vi "串口助手.vi"() -> ()   [LabVIEW 2012]
uses:
  <vilib>/Instr/_visa.llb/VISA Configure Serial Port (Instr).vi
panel:
  in  "复位计数":bool
  in  "接收计数":u32
  in  "发送计数":u32
  in  "清除接收 2":bool
  in  "数据发送":string
  in  "数据接收":string
  in  "清除发送":bool
  in  "清除接收":bool
  in  "循环周期":u32
  in  "循环发送":bool
  in  "文件数据源":bool
  in  "自动附加位":bool
  in  "发送模式":enum32{"ASCII", "HEX"}(radio)
  in  "接收模式":enum32{"ASCII", "HEX"}(radio)
  in  "暂停显示":bool
  in  "文件接收":bool
  in  "接收换行":bool
  in  "日志模式":bool
  in  "停止位":u32(ring)=10 items=["1"=10, "1.5"=15, "2"=20]
  in  "校验位":u16(ring) items=["None", "Odd", "Even", "Mark", "Space"]
  in  "数据位":u16(ring)=8 items=["5"=5, "6"=6, "7"=7, "8"=8]
  in  "波特率":u32(ring)=9600 items=["110"=110, "300"=300, "600"=600, "1200"=1200, "2400"=2400, "4800"=4800, "9600"=9600, "14400"=14400, "19200"=19200, "38400"=38400, "56000"=56000, "57600"=527600, "115200"=115200, "128000"=128000, "256000"=256000]
  in  "串口号":refnum<visa-resource-name>
  in  "打开串口":bool
  # "串口设置"
  # "接收设置"
  # "发送设置"
  # "ms"
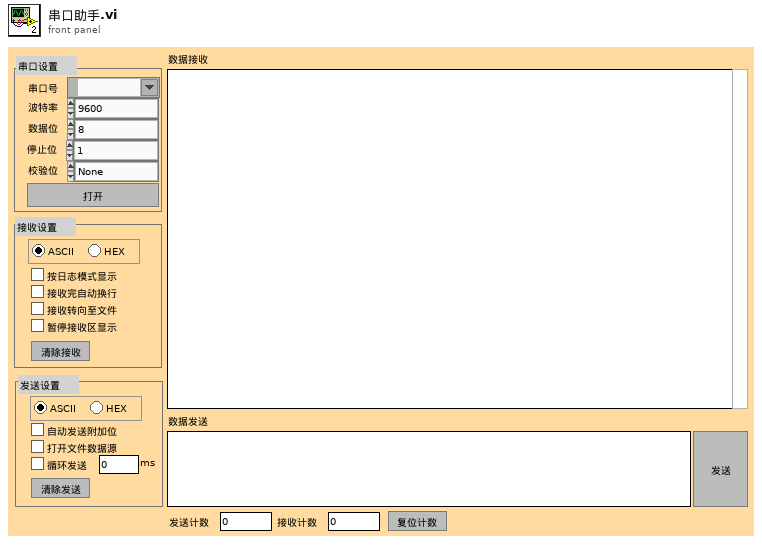
[diagram p1: front panel]
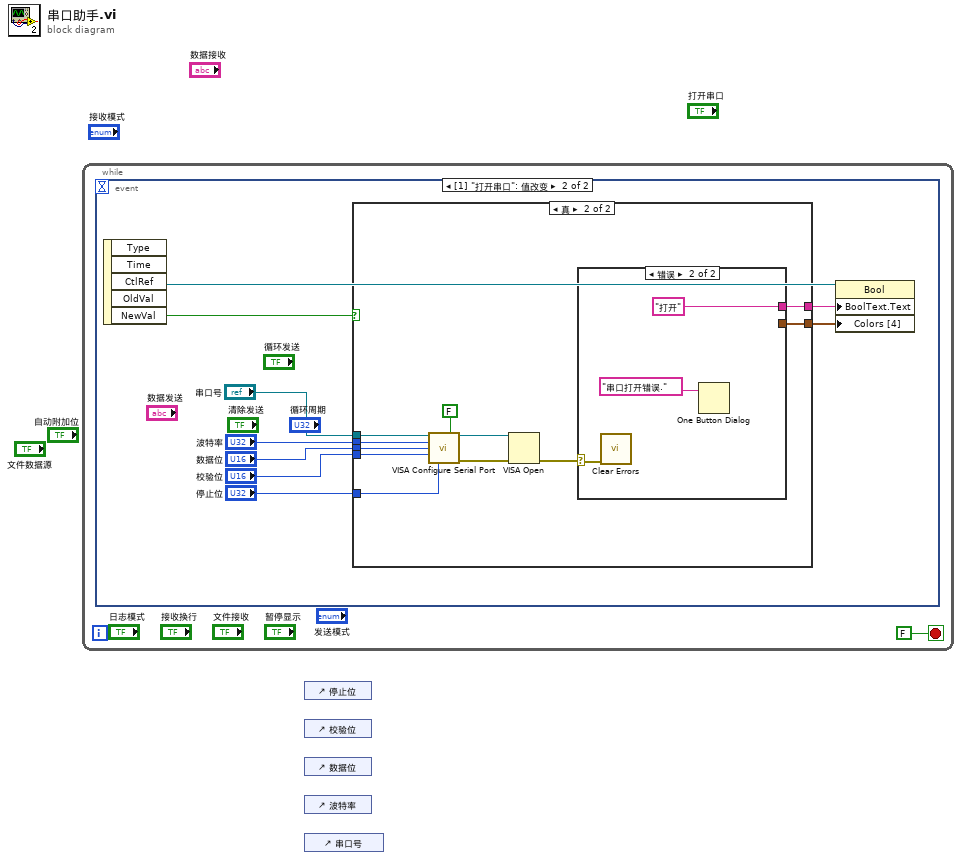
[diagram p0: block diagram]
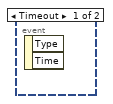
[diagram p2: hidden frame]
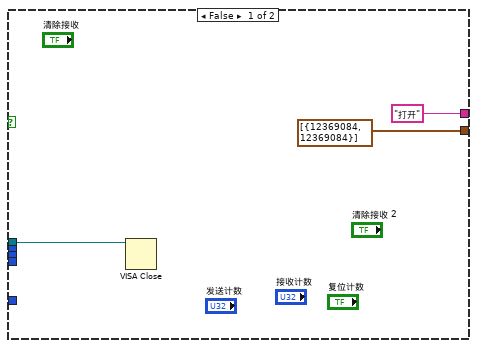
[diagram p3: hidden frame]
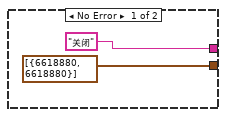
[diagram p4: hidden frame]
diagram:
  n1 = while {
    stop <- FALSE stop-if-true
    n2 = event shown="[1] \"打开串口\": 值改变" {
      selector: _ -> [_ _]
      dyn-events: _ -> [_ _]
      timeout: _ -> [_ _]
      event Timeout {
        n3 = event-data() -> ()  [unwired: 1 in, 2 out]
      }
      event "打开串口": Value Change {
        n4 = event-data() -> ("CtlRef"=w4:refnum<vi>, "NewVal"=w5:bool)  [unwired: 1 in, 3 out]
        n5 = case shown="真" w5 {
          tunnel: "串口号" -> [w13 w23]
          tunnel: "波特率" -> [_ w22]
          tunnel: "数据位" -> [_ w21]
          tunnel: "校验位" -> [_ w20]
          tunnel: "停止位" -> [_ w19]
          tunnel: ["打开" w16] -> w3
          tunnel: [cluster{u32, u32}[] [{12369084, 12369084}] w15] -> w2
          frame False {
            n6 = VISA Close(VISA resource name=w13) -> ()  [unwired: 1 in, 1 out]
          }
          frame True {
            n7 = call-poly "VISA Configure Serial Port"("VISA resource name"=w23, "Enable Termination\nChar (T)"=FALSE ("Enable Termination\nChar (T)"), "baud rate (9600)"=w22, "data bits (8)"=w21, "parity (0:none)"=w20, "stop bits (10: 1 bit)"=w19) -> ("VISA resource name out"=w17:refnum<visa-resource-name>, "error out"=w18:errorcluster)  [unwired: 8 in]
            n8 = VISA Open(error in (no error)=w18, VISA resource name=w17) -> (error out=w14:errorcluster)  [unwired: 3 in, 1 out]
            n9 = case shown="错误" w14 {
              selector: w14 -> [_ w28]
              tunnel: ["关闭" "打开"] -> w16
              tunnel: [cluster{u32, u32}[] [{6618880, 6618880}] _] -> w15
              frame No Error {
              }
              frame Error {
                n10 = call <vilib>:"Clear Errors.vi"("error in (no error)"=w28) -> ()  [unwired: 6 in, 1 out]
                n11 = One Button Dialog(message="串口打开错误.") -> ()  [unwired: 1 in, 1 out]
              }
            }
          }
        }
        n12 = property class="Bool"(reference=w4, "BoolText.Text"=w3, "Colors [4]"=w2) -> ()  [unwired: 1 in, 2 out]
      }
    }
  }
  n13 = control-ref of="停止位"() -> ()  [unwired: 1 out]
  n14 = control-ref of="校验位"() -> ()  [unwired: 1 out]
  n15 = control-ref of="数据位"() -> ()  [unwired: 1 out]
  n16 = control-ref of="波特率"() -> ()  [unwired: 1 out]
  n17 = control-ref of="串口号"() -> ()  [unwired: 1 out]
